vi "Pockels Cal-Condense objectives cal.vi"(11 "Objective power results":string[][](array[string])=[["0", "0", "0", "0"], ["0.1", "", "", ""], ["0.2", "", "6.86", ""], ["0.3", "", "", ""], ["0.4", "37.1", "25.97", "37.1"], ["0.5", "", "", ""], ["0.6", "", "54.39", ""], ["0.7", "", "", ""], ["0.8", "125", "87.5", "125"], ["0.9", "", "", ""], ["1", "", "118.3", ""], ["1.1", "", "", ""], ["1.2", "204", "142.8", "204"], ["1.3", "", "", ""], ["1.4", "", "155.4", ""], ["1.5", "", "", ""], ["1.6", "222", "155.4", "222"], ["1.7", "", "", ""], ["1.8", "", "141.4", ""], ["1.9", "", "", ""], ["2", "152", "106.4", "152"]]) -> (3 "Condensed objective power results":dbl[][](array[numeric]))   [LabVIEW 2020]
uses:
  <userlib>/_OpenG.lib/array/array.llb/Conditional Auto-Indexing Tunnel (Variant)__ogtk.vi
panel:
  out "Condensed objective power results (string)":string[][](array[string])=[["0", "0", "0", "0"], ["0.1", "", "", ""], ["0.2", "", "6.86", ""], ["0.3", "", "", ""], ["0.4", "37.1", "25.97", "37.1"], ["0.5", "", "", ""], ["0.6", "", "54.39", ""], ["0.7", "", "", ""], ["0.8", "125", "87.5", "125"], ["0.9", "", "", ""], ["1", "", "118.3", ""], ["1.1", "", "", ""], ["1.2", "204", "142.8", "204"], ["1.3", "", "", ""], ["1.4", "", "155.4", ""], ["1.5", "", "", ""], ["1.6", "222", "155.4", "222"], ["1.7", "", "", ""], ["1.8", "", "141.4", ""], ["1.9", "", "", ""], ["2", "152", "106.4", "152"]]
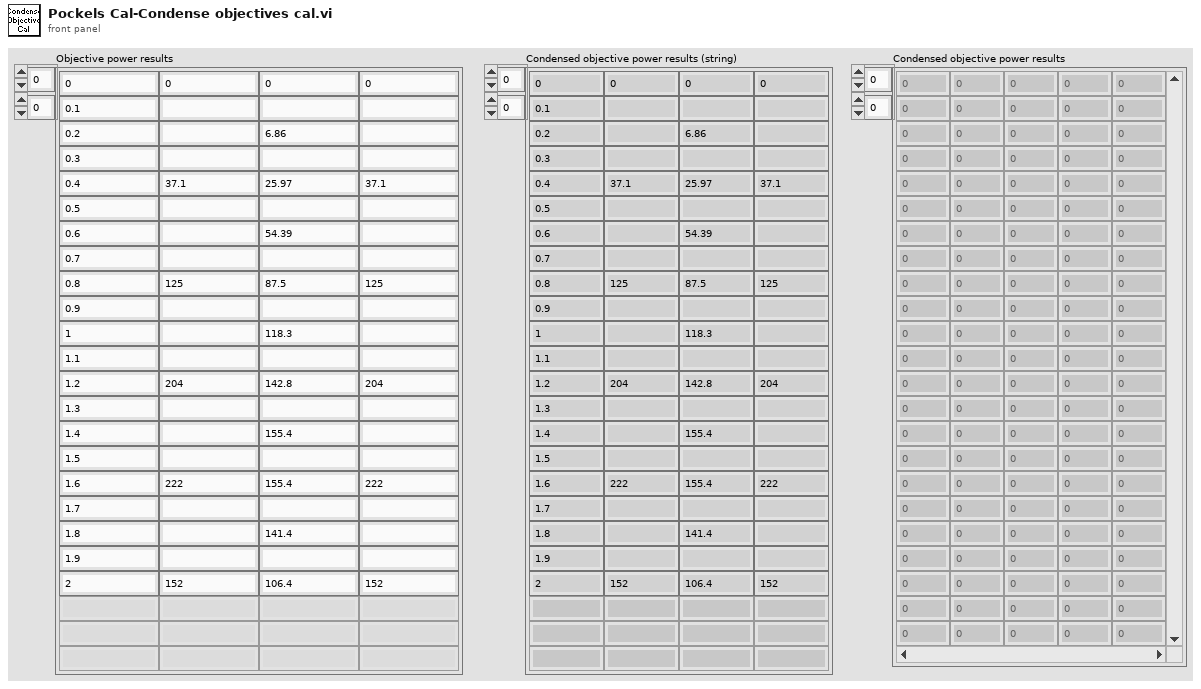
[diagram p1: front panel]
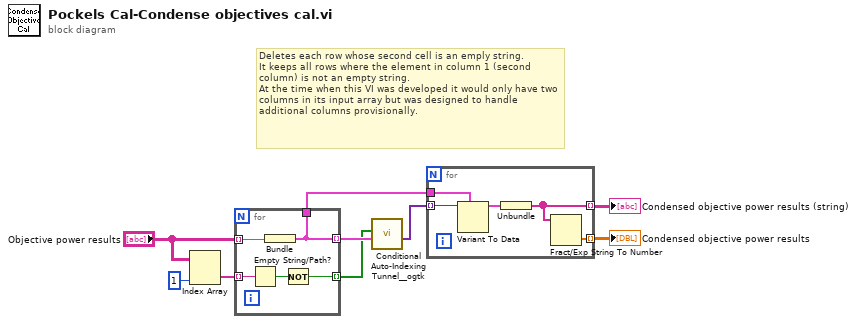
[diagram p0: block diagram]
diagram:
  # "Deletes each row whose second cell is an emply string.\nIt keeps all rows where the element in column 1 (second column) is not an empty string.\nAt the time when this VI was developed it would only have two columns in its input array but was designed to handle additional columns provisionally."
  n1 = Index Array(array="Objective power results", index (col)=1 ("disabled index (col)")) -> (element=w8:string[])  [unwired: 1 in]
  n2 = for {
    tunnel: w8 -> [w14] mode=indexing
    tunnel: [w12] -> w5 mode=indexing
    tunnel: "Objective power results" -> [w11] mode=indexing
    tunnel: [w10] -> w6 mode=indexing
    tunnel: [w10] -> w3
    n3 = Empty String/Path?(string/path=w14) -> (empty?=w13:bool)
    n4 = Bundle("Objective power results"=w11) -> (w10:cluster{"Objective power results":string[]})  [unwired: 1 in]
    n5 = Not(x=w13) -> (.not. x?=w12:bool)
  }
  n6 = call-poly <userlib>:"Conditional Auto-Indexing Tunnel__ogtk.vi"("Array in"=w6, "Elements to keep"=w5) -> ("Filtered Array out"=w4:variant[])  [unwired: 5 in]
  n7 = for {
    tunnel: w4 -> [w18] mode=indexing
    tunnel: w3 -> [w19]
    tunnel: [w16] -> w2 mode=indexing
    tunnel: [w15] -> w1 mode=indexing
    n8 = Variant To Data(type=w19, Variant=w18) -> (data=w17:cluster{"Objective power results":string[]})  [unwired: 1 in, 1 out]
    n9 = Unbundle(w17) -> ("Objective power results"=w16:string[])
    n10 = Fract/Exp String To Number(string=w16) -> (number=w15:dbl[])  [unwired: 3 in, 1 out]
  }
  "Condensed objective power results" <- w1
  "Condensed objective power results (string)" <- w2
